vi "libssh2_knownhost_free.vi"(8 "error in (no error)":errorcluster, 11 "known hosts collection":T1) -> (0 "error out":errorcluster)   [LabVIEW 2013, in "libssh2.lvlib"]
doc: "Frees a collection of known hosts."
uses:
  libssh2.lvlib
  Known Host Collection Refnum.ctl
  Global Settings.vi
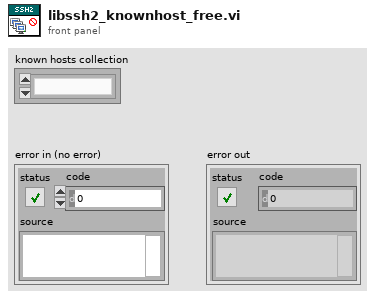
[diagram p1: front panel]
types:
  T1 = typedef "libssh2.lvlib/Known Host Collection Refnum.ctl" = refnum<k1>
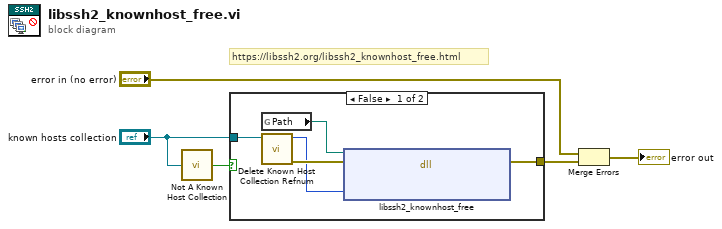
[diagram p0: block diagram]
diagram:
  # "https://libssh2.org/libssh2_knownhost_free.html"
  n1 = call "Not A Known Host Collection.vi"("known hosts collection"="known hosts collection") -> ("Not a Known Hosts Collection?"=w1:bool)
  n2 = case shown="False" w1 {
    tunnel: [w10 _] -> w5
    tunnel: "known hosts collection" -> [w8 _]
    frame False {
      n3 = global read "Global Settings.vi" "Path"() -> (w6:path)
      n4 = call "Delete Known Host Collection Refnum.vi"("known hosts collection"=w8) -> ("error out"=w9:errorcluster, "LIBSSH2_KNOWNHOSTS*"=w7:u64)  [unwired: 9 in]
      n5 = dll-call lib="C:/Users/pasca/source/repos/libssh2-labview/libssh2/libssh2**.*" fn="libssh2_knownhost_free"(path in=w6, error in=w9, "hosts"=w7) -> (error out=w10:errorcluster)  [unwired: 3 in, 1 out]
    }
    frame True {
    }
  }
  n6 = Merge Errors("error in (no error)", w5) -> (→"error out":errorcluster)
